vi "SQL_EDITOR_prepare_INSERT_statement.vi"(8 "error_in":errorcluster, 10 "selected_record":i32, 11 "SQL_EDIT_records":string[][](array[string])) -> (0 "error_out":errorcluster, 3 "INSERT_statement":string)   [LabVIEW 2019]
uses:
  FGV/SQL_EDITOR_records_display/FGV_SQL_EDITOR_records_display.ctl
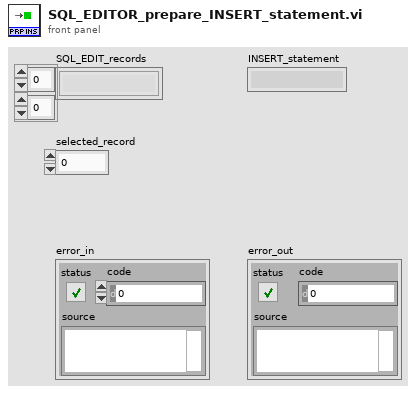
[diagram p1: front panel]
types:
  T1 = typedef "FGV_SQL_EDITOR_records_display.ctl" = enum16{"initialize", "set_table_name", "set_column_name", "set_value_to_select", "set_order_by", "set_asc_desc", "set_headers", "set_records", "get_table_name", "get_column_name", "get_value_to_select", "get_headers", "get_all_info", "record_added?", "record_inserted?", "record_edited?", "record_updated?", "record_deleted?", "discard_changes"}
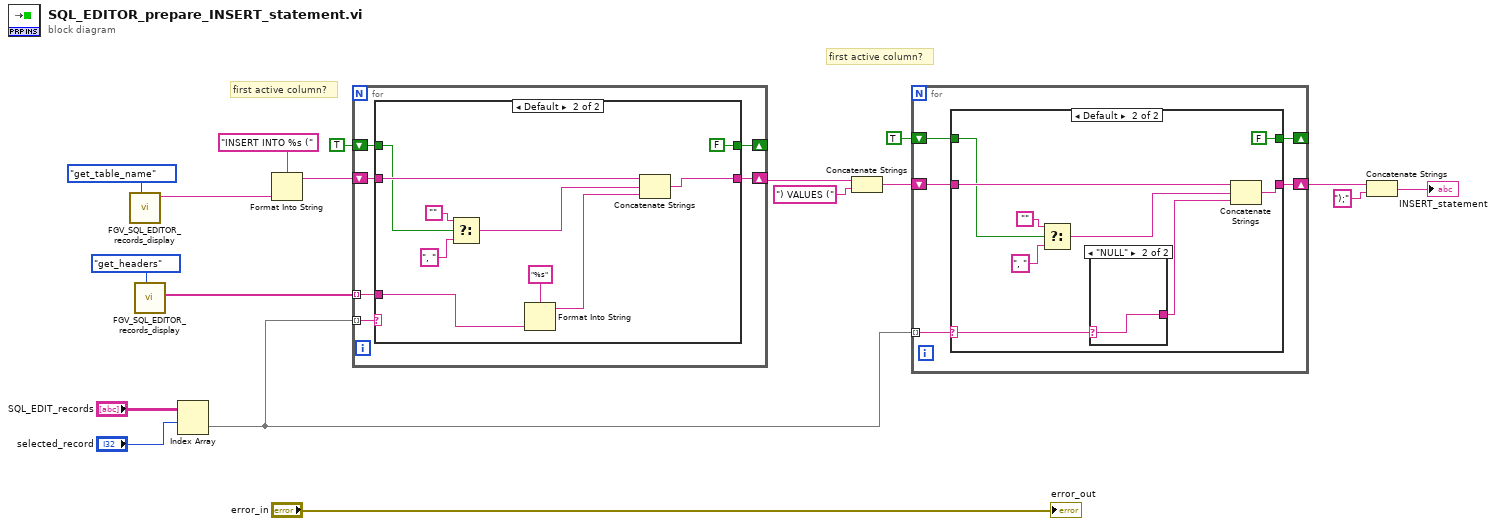
[diagram p0: block diagram]
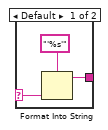
[diagram p3: hidden frame]
diagram:
  # "first active column?"
  # "first active column?"
  n1 = call "FGV_SQL_EDITOR_records_display.vi"("options"=FGV_SQL_EDITOR_records_display."get_table_name") -> ("string_param_output"=w6:string)  [unwired: 7 in, 3 out]
  n2 = call "FGV_SQL_EDITOR_records_display.vi"("options"=FGV_SQL_EDITOR_records_display."get_headers") -> ("array_param_output"=w5:string[])  [unwired: 7 in, 3 out]
  n3 = Index Array(array="SQL_EDIT_records", index (row)="selected_record") -> (element=w1:string[])  [unwired: 1 in]
  n4 = Format Into String(format string="INSERT INTO %s (", w6) -> (resulting string=w13:string)  [unwired: 2 in, 1 out]
  n5 = for {
    tunnel: w5 -> [w22] mode=indexing
    shift-right: [w23] -> w15
    shift-left: w13 -> [w24]
    shift-right: [w19] -> _
    shift-left: TRUE -> [w21]
    tunnel: w1 -> [w20] mode=indexing
    n6 = case shown="Default" w20 {
      tunnel: w24 -> [w25 w34]
      tunnel: [w25 w33] -> w23
      tunnel: w22 -> [_ w31]
      tunnel: w21 -> [w26 w28]
      tunnel: [w26 FALSE] -> w19
      frame "" {
      }
      frame Default {
        n7 = Select(t="", s=w28, f=", ") -> (s? t:f=w32:string)
        n8 = Format Into String(format string="%s", w31) -> (resulting string=w30:string)  [unwired: 2 in, 1 out]
        n9 = Concatenate Strings(w34, w32, w30) -> (w33:string)
      }
    }
  }
  n10 = Concatenate Strings(w15, ") VALUES (" ("string")) -> (w11:string)
  n11 = for {
    tunnel: w1 -> [w39] mode=indexing
    shift-right: [w40] -> w9
    shift-left: w11 -> [w41]
    shift-right: [w37] -> _
    shift-left: TRUE -> [w38]
    n12 = case shown="Default" w39 {
      selector: w39 -> [_ w47]
      tunnel: w41 -> [w43 w50]
      tunnel: [w43 w49] -> w40
      tunnel: w38 -> [w42 w44]
      tunnel: [w42 FALSE] -> w37
      frame "" {
      }
      frame Default {
        n13 = Select(t="", s=w44, f=", ") -> (s? t:f=w48:string)
        n14 = case shown="\"NULL\"" w47 {
          selector: w47 -> [w55 w56]
          tunnel: [w54 w56] -> w46
          frame Default {
            n15 = Format Into String(format string="'%s'", w55) -> (resulting string=w54:string)  [unwired: 2 in, 1 out]
          }
          frame "NULL" {
          }
        }
        n16 = Concatenate Strings(w50, w48, w46) -> (w49:string)
      }
    }
  }
  n17 = Concatenate Strings(w9, ");" ("string")) -> (→"INSERT_statement":string)
  "error_out" <- "error_in"
